vi "M04 Solar Farm.vi"(11 "EV3 in":T1) -> ()   [LabVIEW 2016]
uses:
  <vilib>/NXT/Subs/LVHSConnector.ctl
  <vilib>/NXT/LegoClasses/BrickReference/BrickReference.lvclass
  <vilib>/NXT/Block Support/NXT_OutputPort.ctl
  <vilib>/NXT/NXTIO Xnodes/NXTIONodeSubVIs/LEGOResetMotors.vi
  <vilib>/NXT/NXTIO Xnodes/NXTIONodeSubVIs/NXTMotorRunDistance.vi
  <vilib>/NXT/NXTIO Xnodes/AddressXNode/NXTIOAddress.xnode
  <vilib>/NXT/NXTIO Xnodes/NXTIOXNode/NXTIO.xnode
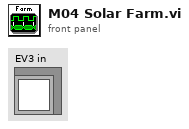
[diagram p1: front panel]
types:
  T1 = typedef "LVHSConnector.ctl" = refnum<class "BrickReference.lvclass">
  T2 = typedef "NXT_OutputPort.ctl" = u8
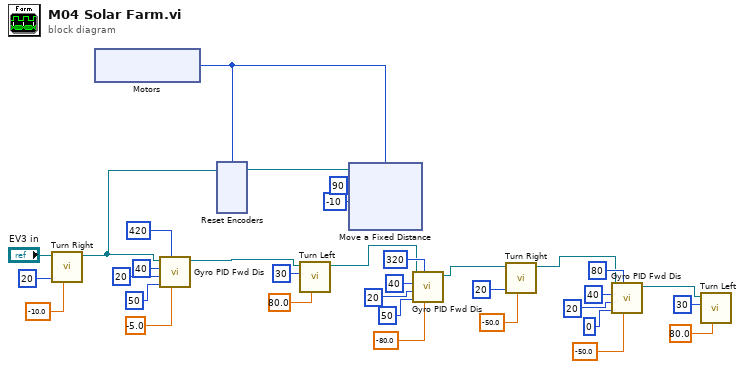
[diagram p0: block diagram]
diagram:
  n1 = call "Turn Right.vi"("Turning angle"=sgl -10.0, "Motor B (right)"=i8 20, "EV3 in"="EV3 in") -> ("EV3 out"=w22:T1)  [unwired: 8 in]
  n2 = xnode "Motors"() -> ("Motor"=w23:T2)
  n3 = call "Gyro PID Fwd Dis.vi"("Target angle"=sgl -5.0, "Threshold to stop"=420, "Threshold to slow"=50, "Min. speed"=20, "Max. speed"=40, "EV3 in"=w22) -> ("EV3 out"=w19:T1)  [unwired: 5 in]
  n4 = xnode "Reset Encoders"("Motors"=w23, "NXT/EV3"=w22) -> ("NXT/EV3"=w24:T1)
  n5 = call "Turn Left.vi"("Turning angle"=sgl 80.0, "Motor B (right)"=i8 30, "EV3 in"=w19) -> ("EV3 out"=w14:T1)  [unwired: 8 in]
  n6 = xnode "Move a Fixed Distance"("Speed 1"=i8 -10, "Distance 1"=90, "Motors"=w23, "NXT/EV3"=w24) -> ()  [unwired: 1 out]
  n7 = call "Gyro PID Fwd Dis.vi"("Target angle"=sgl -80.0, "Threshold to stop"=320, "Threshold to slow"=50, "Min. speed"=20, "Max. speed"=40, "EV3 in"=w14) -> ("EV3 out"=w10:T1)  [unwired: 5 in]
  n8 = call "Turn Right.vi"("Turning angle"=sgl -50.0, "Motor B (right)"=i8 20, "EV3 in"=w10) -> ("EV3 out"=w4:T1)  [unwired: 8 in]
  n9 = call "Gyro PID Fwd Dis.vi"("Target angle"=sgl -50.0, "Threshold to stop"=80, "Threshold to slow"=0, "Min. speed"=20, "Max. speed"=40, "EV3 in"=w4) -> ("EV3 out"=w1:T1)  [unwired: 5 in]
  n10 = call "Turn Left.vi"("Turning angle"=sgl 80.0, "Motor B (right)"=i8 30, "EV3 in"=w1) -> ()  [unwired: 8 in, 1 out]
